vi "Controller - Input Messages.vi"(8 "error in (no error)":errorcluster, 11 "FilePath":path) -> (0 "error out":errorcluster, 3 "Messages":string[](array[string]))   [LabVIEW 2017]
doc: "Reads all messages of ATM controllerfrom external file."
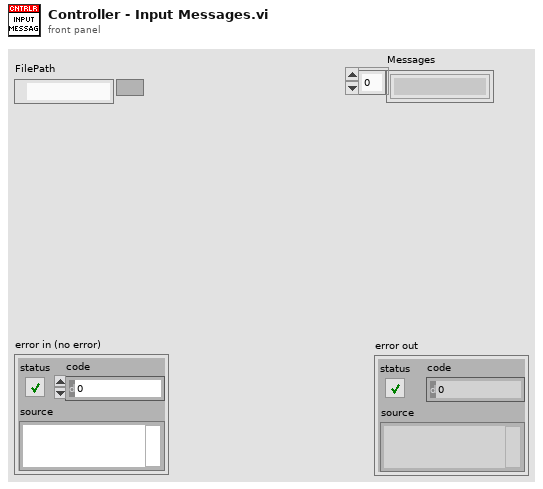
[diagram p1: front panel]
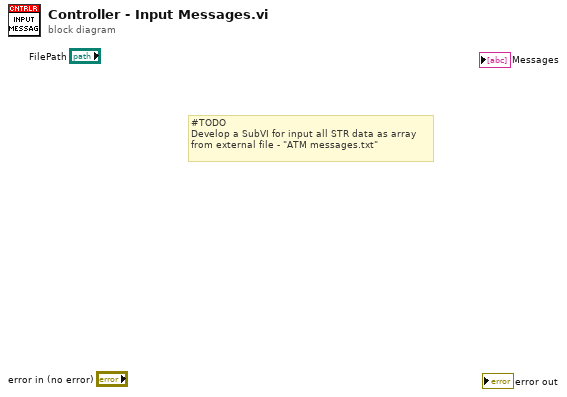
[diagram p0: block diagram]
diagram:
  # "#TODO\nDevelop a SubVI for input all STR data as array\nfrom external file - \"ATM messages.txt\""
